vi "IMU2JointAnglesAdv.vi"(6 "Operation(GetData)":T1, 7 "JointAngleDir([-1,1,1,-1])":dbl[](array[numeric])=[-1.0, 1.0, 1.0, -1.0], 8 "error in (no error)":errorcluster, 11 "IMU in (rad)":dbl[][](array[numeric])) -> (0 "error out":errorcluster, 3 "Joint Angles (rad)":dbl[](array[numeric]))   [LabVIEW 2016]
uses:
  TypeDef/IMU_operation.ctl
  <vilib>/imath/engines/lvmath2/RunTimeEngine/NodeEndStatement/NIMS_NodeEndStatement_Output.vi
  <instcachedir>/0/NIMS_NodeEndStatement_Output_53EC0D466D134D7ABD903AC30B43404B.lvgen/NIMS_NodeEndStatement_Output_53EC0D466D134D7ABD903AC30B43404B_001.vi
  <vilib>/imath/engines/lvmath2/RunTimeEngine/ErrorHandling/NIMS_Finalize Error.vi
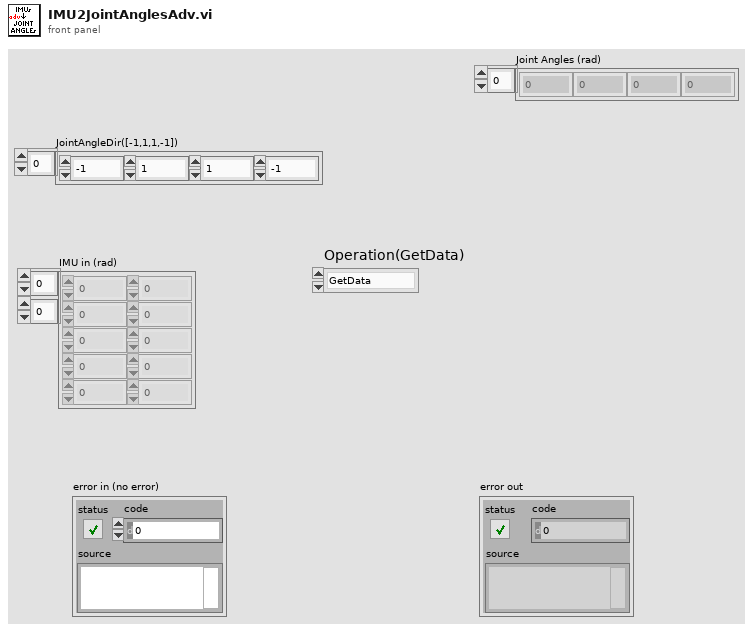
[diagram p1: front panel]
types:
  T1 = typedef "IMU_operation.ctl" = enum16{"GetData", "ClearStandPos", "SetStandPos"}
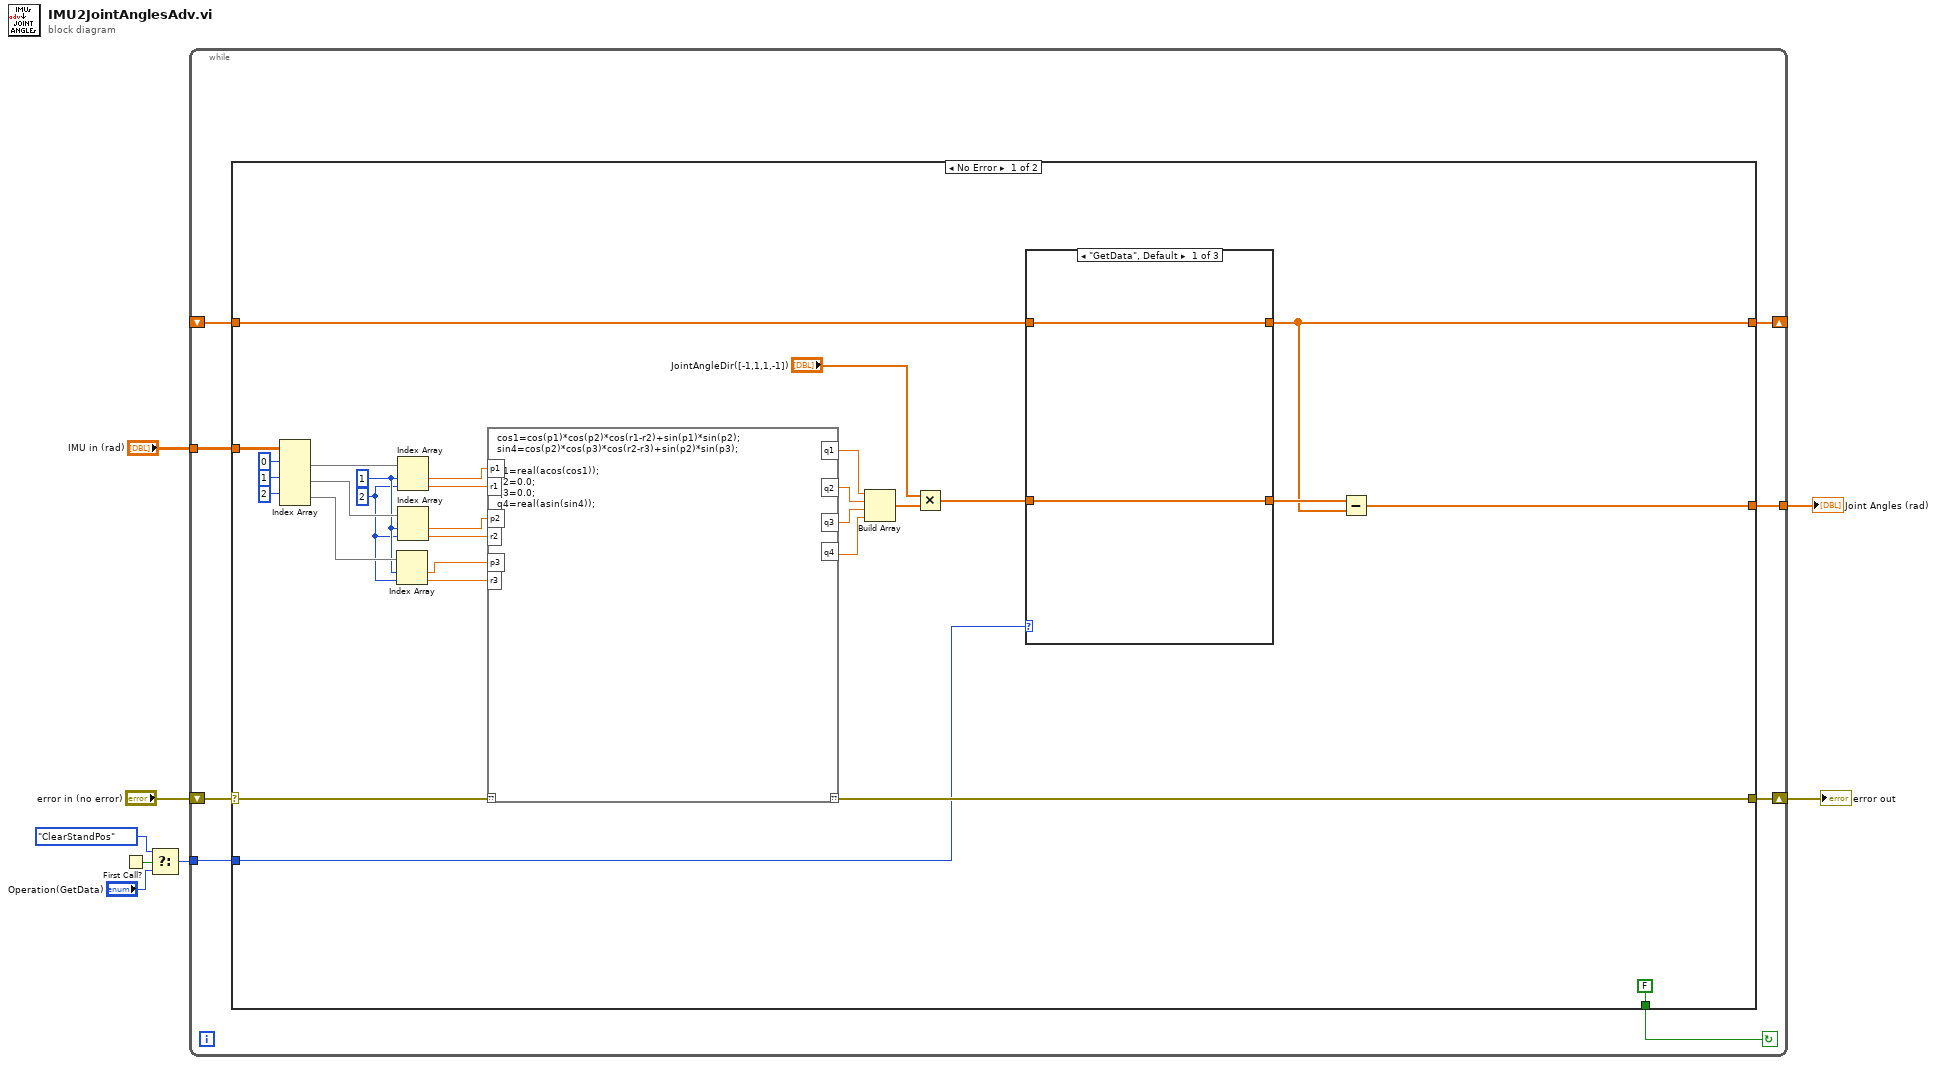
[diagram p0: block diagram]
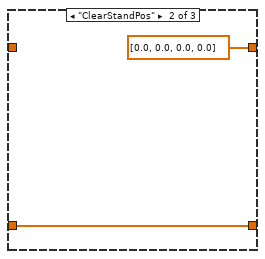
[diagram p2: hidden frame]
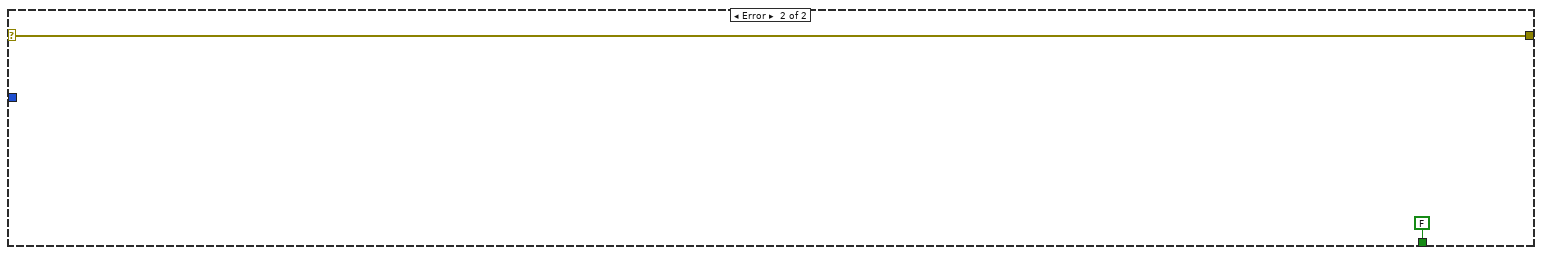
[diagram p4: hidden frame]
diagram:
  n1 = First Call?() -> (First Call?: T/F=w4:bool)
  n2 = Select(t=IMU_operation."ClearStandPos", s=w4, f="Operation(GetData)") -> (s? t:f=w2:T1)
  n3 = while {
    tunnel: [w16] -> w8
    tunnel: "IMU in (rad)" -> [w15]
    shift-right: [w13] -> w5
    shift-left: "error in (no error)" -> [w14]
    tunnel: w2 -> [w11]
    shift-right: [w10] -> _
    shift-left: _ -> [w9]
    stop <- w12 continue-if-true
    n4 = case shown="No Error" w14 {
      selector: w14 -> [w31 w141]
      tunnel: [w18 _] -> w16
      tunnel: w15 -> [w43 _]
      tunnel: [w30 w141] -> w13
      tunnel: [FALSE FALSE] -> w12
      tunnel: w11 -> [w24 _]
      tunnel: [w19 _] -> w10
      tunnel: w9 -> [w22 _]
      frame No Error {
        w38 = 2 ("index")
        w39 = 1 ("index")
        n5 = Index Array(array=w43, index (row) #1=0 ("index (row)"), index (row) #2=1 ("index (row)"), index (row) #3=2 ("index (row)")) -> (element #1=w42:dbl[], element #2=w41:dbl[], element #3=w40:dbl[])  [unwired: 3 in]
        n6 = Index Array(array=w40, index #1=w39, index #2=w38) -> (element #1=w33:dbl, element #2=w32:dbl)
        n7 = Index Array(array=w42, index #1=w39, index #2=w38) -> (element #1=w37:dbl, element #2=w36:dbl)
        n8 = Index Array(array=w41, index #1=w39, index #2=w38) -> (element #1=w35:dbl, element #2=w34:dbl)
        n9 = mathscript code="cos1=cos(p1)*cos(p2)*cos(r1-r2)+sin(p1)*sin(p2);\nsin4=cos(p2)*cos(p3)*cos(r2-r3)+sin(p2)*sin(p3);\n\nq1=real(acos(cos1));\nq2=0.0;\nq3=0.0;\nq4=real(asin(sin4));"("??"=w31, "p1"=w37, "r1"=w36, "p2"=w35, "r2"=w34, "p3"=w33, "r3"=w32) -> ("??"=w30:errorcluster, "q1"=w23:dbl, "q2"=w27:dbl, "q3"=w28:dbl, "q4"=w29:dbl)
        n10 = Build Array(w23, w27, w28, w29) -> (w25:dbl[])
        n11 = Multiply(x="JointAngleDir([-1,1,1,-1])", y=w25) -> (x*y=w21:dbl[])
        n12 = case shown="\"GetData\", Default" w24 {
          tunnel: [w48 dbl[] [0.0, 0.0, 0.0, 0.0] w51] -> w19
          tunnel: w22 -> [w48 _ _]
          tunnel: w21 -> [w47 w49 w51]
          tunnel: [w47 w49 w51] -> w20
          frame "GetData", Default {
          }
          frame "ClearStandPos" {
          }
          frame "SetStandPos" {
          }
        }
        n13 = Subtract(x=w20, y=w19) -> (x-y=w18:dbl[])
      }
      frame Error {
      }
    }
  }
  "Joint Angles (rad)" <- w8
  "error out" <- w5
